vi "Create Filename.vi"(8 "error in":errorcluster, 10 "Path in":path=path "C:/Projects/Data", 11 "Data in":T1={"session"=refnum, "IsOpen"=FALSE, "Timeout (ms)"=0, "TempFile"=path "", "LogStartTime"=timestamp(0 s since 1904-01-01), "LibreVNA"=refnum, "VNAOpen"=FALSE, "TempSP"=0.0, "ActualTemp"=0.0, "FileSaved"=FALSE, "PIDOutput"=0.0, "VNALogOpt"=refnum, "PartName"="PartNumber1", "ComPort"="", "S-Param Data"=[], "VNADataFile - TDMS"=path ""} {"LogStartTime" format="%<%x %.3X>T"}) -> (0 "error out":errorcluster, 1 "TDMS FileName":path, 3 "Data Out":T1 {"LogStartTime" format="%<%x %.3X>T"})   [LabVIEW 2023]
uses:
  controls/UI Data.ctl
  <vilib>/NI/Modbus Library/API/Master/Modbus Master.lvclass
  LibreVNA/LibreVNA.lvclass
  <vilib>/Utility/error.llb/Trim Whitespace One-Sided.vi
  <vilib>/Utility/file.llb/Write Delimited Spreadsheet (string).vi
panel:
  out "TempFile":path
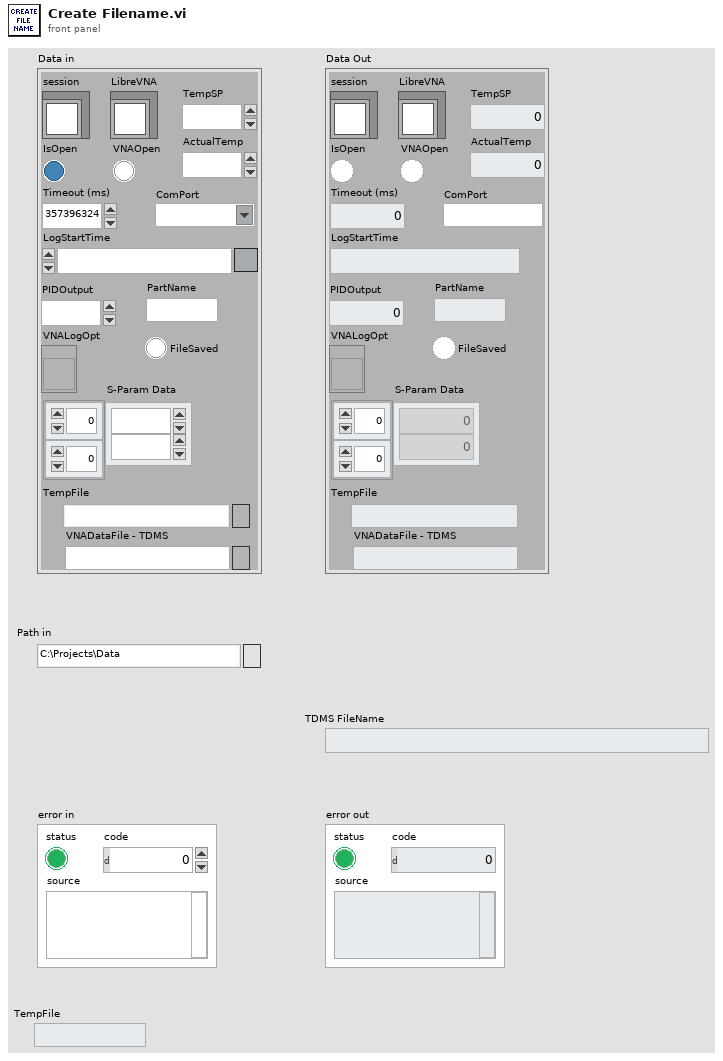
[diagram p1: front panel]
types:
  T1 = typedef "UI Data.ctl" = cluster{"session":refnum<class "Modbus Master.lvclass">, "IsOpen":bool, "Timeout (ms)":i32, "TempFile":path, "LogStartTime":timestamp, "LibreVNA":refnum<class "LibreVNA.lvclass">, "VNAOpen":bool, "TempSP":dbl, "ActualTemp":dbl, "FileSaved":bool, "PIDOutput":dbl, "VNALogOpt":refnum<vi>, "PartName":string, "ComPort":refnum<visa-resource-name>, "S-Param Data":dbl[][], "VNADataFile - TDMS":path}
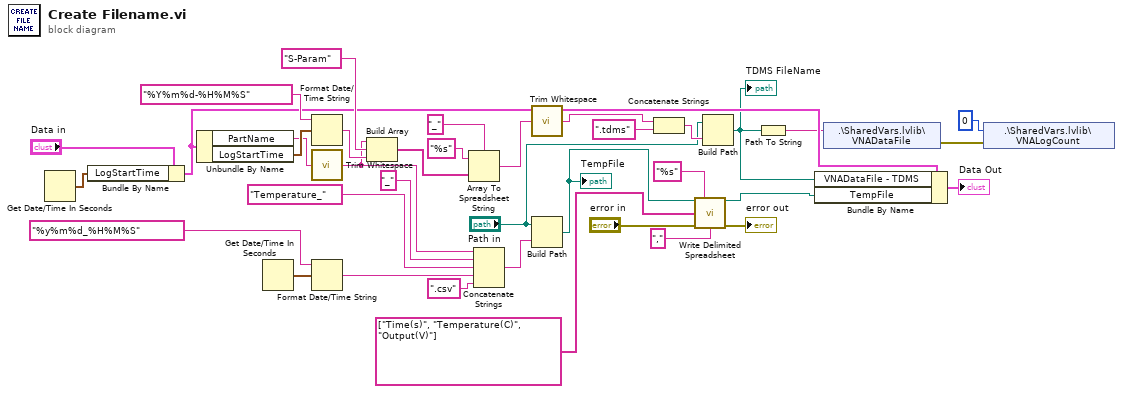
[diagram p0: block diagram]
diagram:
  n1 = Get Date/Time In Seconds() -> (seconds since 1Jan1904=w20:timestamp)
  n2 = Bundle By Name(cluster="Data in", "LogStartTime"=w20) -> (w21:T1)
  n3 = Unbundle By Name(w21) -> ("PartName"=w23:string, "LogStartTime"=w28:timestamp)
  n4 = Get Date/Time In Seconds() -> (seconds since 1Jan1904=w12:timestamp)
  n5 = Format Date/Time String(time format string (%c)="%Y%m%d-%H%M%S", seconds (now)=w28) -> (date/time string=w34:string)  [unwired: 1 in]
  n6 = call <vilib>:"Trim Whitespace.vi"("string"=w23) -> ("trimmed string"=w10:string)  [unwired: 1 in]
  n7 = Format Date/Time String(time format string (%c)="%y%m%d_%H%M%S", seconds (now)=w12) -> (date/time string=w16:string)  [unwired: 1 in]
  n8 = Build Array(w10, "S-Param" ("element"), w34) -> (w33:string[])
  n9 = Array To Spreadsheet String(delimiter (Tab)="_", array=w33, 3:"%s" ("format string")) -> (spreadsheet string=w30:string)
  n10 = Concatenate Strings(w10, "_" ("string"), "Temperature_" ("string"), w16, ".csv" ("string")) -> (w13:string)
  n11 = call <vilib>:"Trim Whitespace.vi"("string"=w30) -> ("trimmed string"=w27:string)  [unwired: 1 in]
  n12 = Build Path(base path="Path in", name or relative path=w13) -> (appended path=w7:path)
  "TempFile" <- w7
  n13 = Concatenate Strings(w27, ".tdms" ("string")) -> (w25:string)
  n14 = call-poly <vilib>:"Write Delimited Spreadsheet.vi"("file path (dialog if empty)"=w7, "format (%s)"="%s", "1D data"=string[] ["Time(s)", "Temperature(C)", "Output(V)"], "error in (no error)"="error in", "delimiter (\\t)"="," ("delimiter (\\t)")) -> ("new file path (Not A Path if cancelled)"=w6:path, "error out"=→"error out":errorcluster)  [unwired: 9 in]
  n15 = Build Path(base path="Path in", name or relative path=w25) -> (appended path=w3:path)
  "TDMS FileName" <- w3
  n16 = Path To String(path=w3) -> (string=w2:string)
  n17 = Bundle By Name(cluster=w21, "VNADataFile - TDMS"=w3, "TempFile"=w6) -> (→"Data Out":T1)
  n18 = shared-variable ".\\SharedVars.lvlib\\VNADataFile"(w2) -> (error out=w1:errorcluster)  [unwired: 1 in]
  n19 = shared-variable ".\\SharedVars.lvlib\\VNALogCount"(u32 0 ("VNALogCount"), error in=w1) -> ()  [unwired: 1 out]
